vi "Read Swipe.vi"   [LabVIEW 2011, in "LMH-Leap.lvlib"]
doc: "Read all data from swipe gestures. Use the polymorphic instance to select between one and N swipe gestures."
uses:
  LMH-Leap.lvlib
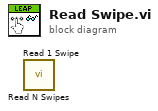
[diagram p0: block diagram]
diagram:
  n1 = call "Read N Swipes.vi"() -> ()  [unwired: 8 in, 4 out]
  n2 = call "Read 1 Swipe.vi"() -> ()  [unwired: 8 in, 4 out]
